vi "Resize Subpanel.vi"(8 "error in (no error)":errorcluster, 10 "Subpanel Size":T1, 11 "UI Controller in":refnum<class "UI Controller.lvclass">) -> (0 "error out":errorcluster, 3 "UI Controller out":refnum<class "UI Controller.lvclass">)   [LabVIEW 2020, in "UI Controller.lvlib" / "UI Controller.lvclass"]
uses:
  UI Controller.lvclass
  C:/Program Files/National Instruments/LabVIEW 2020/vi.lib/ActorFrameworkMVC/View Controller/View Controller/View Controller.lvclass
  <vilib>/Utility/miscctls.llb/LVBoundsTypeDef.ctl
  <vilib>/ActorFrameworkMVC/View Controller/View Controller/View Controller.lvclass
panel:
  # "NOTICE -- YOU MUST LEAVE THIS NOTICE IN PLACE.\n\nCopyright (c) 2017, LIANG LIU Shawn.Liu.cn@gmail.com\nAll rights reserved.\n\nRedistribution and use in source and binary forms, with or without modification, are permitted provided that the following conditions are met:\n-Redistributions of source code must retain the above copyright notice, this list of conditions and the following disclaimer.\n-Redistributions in binary form must reproduce the above copyright notice, this list of conditions and the following disclaimer in the documentation and/or other materials provided with the distribution.\n-Neither the name of the eLp nor the names of its contributors may be used to endorse or promote products derived from this software without specific prior written permission.\n\nTHIS SOFTWARE IS PROVIDED BY THE COPYRIGHT HOLDERS AND CONTRIBUTORS \"AS IS\" AND ANY EXPRESS OR IMPLIED WARRANTIES, INCLUDING, BUT NOT LIMITED TO, THE IMPLIED WARRANTIES OF MERCHANTABILITY AND FITNESS FOR A PARTICULAR PURPOSE ARE DISCLAIMED. IN NO EVENT SHALL THE COPYRIGHT HOLDER OR CONTRIBUTORS BE LIABLE FOR ANY DIRECT, INDIRECT, INCIDENTAL, SPECIAL, EXEMPLARY, OR CONSEQUENTIAL DAMAGES (INCLUDING, BUT NOT LIMITED TO, PROCUREMENT OF SUBSTITUTE GOODS OR SERVICES; LOSS OF USE, DATA, OR PROFITS; OR BUSINESS INTERRUPTION) HOWEVER CAUSED AND ON ANY THEORY OF LIABILITY, WHETHER IN CONTRACT, STRICT LIABILITY, OR TORT (INCLUDING NEGLIGENCE OR OTHERWISE) ARISING IN ANY WAY OUT OF THE USE OF THIS SOFTWARE, EVEN IF ADVISED OF THE POSSIBILITY OF SUCH DAMAGE."
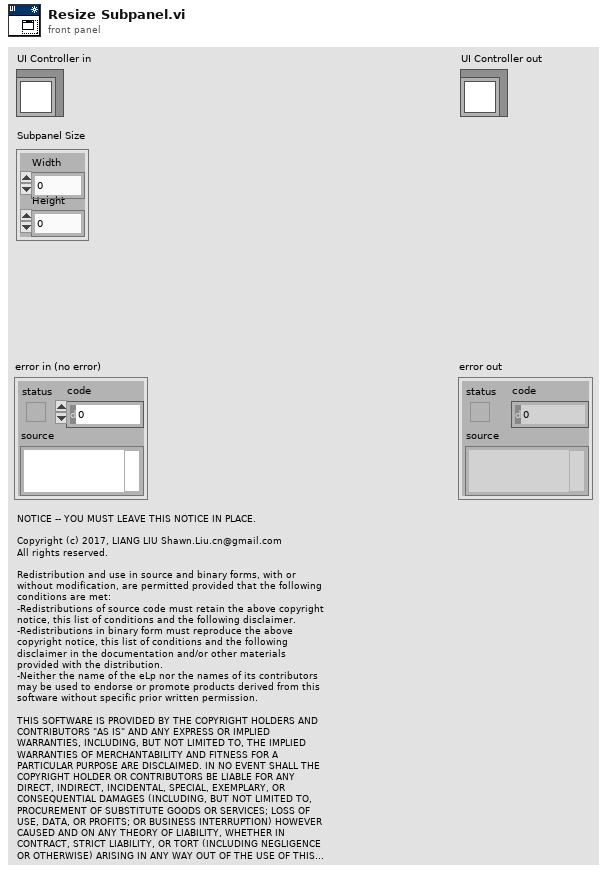
[diagram p1: front panel]
types:
  T1 = typedef "LVBoundsTypeDef.ctl" = cluster{"Width":u32, "Height":u32}
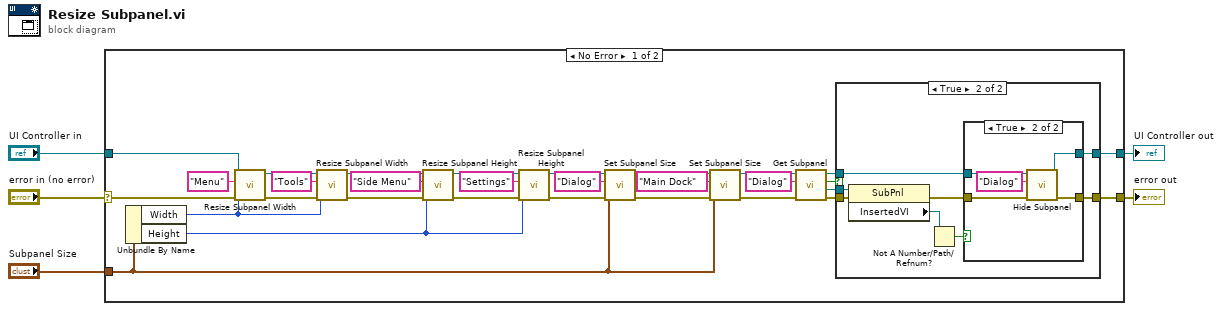
[diagram p0: block diagram]
diagram:
  n1 = case shown="No Error" "error in (no error)" {
    selector: "error in (no error)" -> [w34 w54]
    tunnel: "UI Controller in" -> [w35 w53]
    tunnel: [w14 w54] -> w3
    tunnel: "Subpanel Size" -> [w7 _]
    tunnel: [w6 w53] -> w1
    frame No Error {
      n2 = Unbundle By Name(w7) -> ("Width"=w23:u32, "Height"=w22:u32)
      n3 = call "Resize Subpanel Width.vi"("error in (no error)"=w34, "Width"=w23, "Subpanel Name"="Menu", "UI Controller in"=w35) -> ("error out"=w26:errorcluster, "UI Controller out"=w30:refnum<class "UI Controller.lvclass">)  [unwired: 6 in]
      n4 = call "Resize Subpanel Width.vi"("error in (no error)"=w26, "Width"=w23, "Subpanel Name"="Tools", "UI Controller in"=w30) -> ("error out"=w25:errorcluster, "UI Controller out"=w29:refnum<class "UI Controller.lvclass">)  [unwired: 6 in]
      n5 = call "Resize Subpanel Height.vi"("error in (no error)"=w25, "Height"=w22, "Subpanel Name"="Side Menu", "UI Controller in"=w29) -> ("error out"=w24:errorcluster, "UI Controller out"=w33:refnum<class "UI Controller.lvclass">)  [unwired: 6 in]
      n6 = call "Resize Subpanel Height.vi"("error in (no error)"=w24, "Height"=w22, "Subpanel Name"="Settings", "UI Controller in"=w33) -> ("error out"=w12:errorcluster, "UI Controller out"=w13:refnum<class "UI Controller.lvclass">)  [unwired: 6 in]
      n7 = call <vilib>:"Set Subpanel Size.vi"("error in (no error)"=w12, "Subpanel Size"=w7, "Subpanel Name"="Dialog", "View Controller in"=w13) -> ("error out"=w10:errorcluster, "View Controller out"=w11:refnum<class "UI Controller.lvclass">)  [unwired: 5 in, 1 out]
      n8 = call <vilib>:"Set Subpanel Size.vi"("error in (no error)"=w10, "Subpanel Size"=w7, "Subpanel Name"="Main Dock", "View Controller in"=w11) -> ("error out"=w8:errorcluster, "View Controller out"=w9:refnum<class "UI Controller.lvclass">)  [unwired: 5 in, 1 out]
      n9 = call <vilib>:"Get Subpanel.vi"("error in (no error)"=w8, "Subpanel Name"="Dialog", "View Controller in"=w9) -> ("error out"=w20:errorcluster, "Subpanel Reference"=w16:refnum<vi>, "Found?"=w17:bool, "View Controller out"=w19:refnum<class "UI Controller.lvclass">)  [unwired: 5 in]
      n10 = case shown="True" w17 {
        tunnel: [w37 w39] -> w14
        tunnel: w20 -> [w37 w45]
        tunnel: w19 -> [w36 w44]
        tunnel: w16 -> [_ w42]
        tunnel: [w36 w38] -> w6
        frame False {
        }
        frame True {
          n11 = property class="SubPnl"(reference=w42, error in=w45) -> (error out=w43:errorcluster, "InsertedVI"=w41:refnum<vi>)  [unwired: 1 out]
          n12 = Not A Number/Path/Refnum?(number/path/refnum=w41) -> (NaN/Path/Refnum?=w40:bool)
          n13 = case shown="True" w40 {
            tunnel: [w47 w52] -> w39
            tunnel: w44 -> [w46 w48]
            tunnel: w43 -> [w47 w51]
            tunnel: [w46 w49] -> w38
            frame False {
            }
            frame True {
              n14 = call "Hide Subpanel.vi"("error in (no error)"=w51, "Subpanel Name"="Dialog", "UI Controller in"=w48) -> ("error out"=w52:errorcluster, "UI Controller out"=w49:refnum<class "UI Controller.lvclass">)  [unwired: 7 in]
            }
          }
        }
      }
    }
    frame Error {
    }
  }
  "error out" <- w3
  "UI Controller out" <- w1
